vi "Semaphore.vi"() -> ()   [LabVIEW 2020]
panel:
  out "Read":i32
  out "Write":i32
  in  "stop":bool
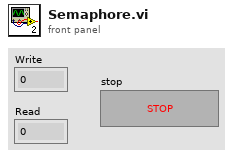
[diagram p1: front panel]
types:
  T1 = typedef "Semaphore RefNum" = refnum<k1>
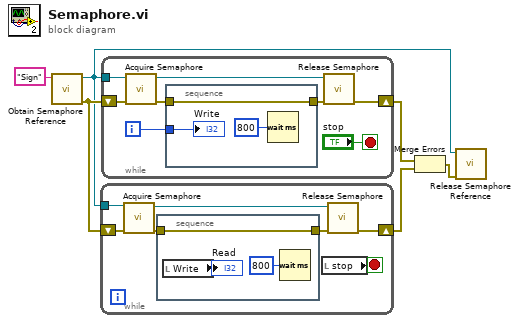
[diagram p0: block diagram]
diagram:
  n1 = call <vilib>:"Obtain Semaphore Reference.vi"("name (unnamed)"="Sign") -> ("error out"=w5:errorcluster, "semaphore"=w4:T1)  [unwired: 4 in, 1 out]
  n2 = while {
    tunnel: w4 -> [w13]
    shift-right: [w7] -> w2
    shift-left: w5 -> [w12]
    stop <- w11 stop-if-true
    n3 = call <vilib>:"Acquire Semaphore.vi"("error in (no error)"=w12, "semaphore"=w13) -> ("error out"=w10:errorcluster, "semaphore out"=w8:T1)  [unwired: 3 in, 1 out]
    n4 = stacked-sequence {
      tunnel: [w16] -> w9
      tunnel: w10 -> [w16]
      frame #0 {
        n5 = local read "Write"() -> (→"Read":i32)
        n6 = Wait (ms)(milliseconds to wait=u32 800) -> ()  [unwired: 1 out]
      }
    }
    n7 = local read "stop"() -> (w11:bool)
    n8 = call <vilib>:"Release Semaphore.vi"("error in (no error)"=w9, "semaphore"=w8) -> ("error out"=w7:errorcluster)  [unwired: 4 in, 1 out]
  }
  n9 = while {
    tunnel: w4 -> [w24]
    shift-right: [w17] -> w3
    shift-left: w5 -> [w23]
    i -> [w19]
    stop <- "stop" stop-if-true
    n10 = call <vilib>:"Acquire Semaphore.vi"("error in (no error)"=w23, "semaphore"=w24) -> ("error out"=w21:errorcluster, "semaphore out"=w18:T1)  [unwired: 3 in, 1 out]
    n11 = stacked-sequence {
      tunnel: w21 -> [w27]
      tunnel: [w27] -> w20
      tunnel: w19 -> [w26]
      frame #0 {
        n12 = Wait (ms)(milliseconds to wait=u32 800) -> ()  [unwired: 1 out]
        "Write" <- w26
      }
    }
    n13 = call <vilib>:"Release Semaphore.vi"("error in (no error)"=w20, "semaphore"=w18) -> ("error out"=w17:errorcluster)  [unwired: 4 in, 1 out]
  }
  n14 = Merge Errors(w3, w2) -> (w1:errorcluster)
  n15 = call <vilib>:"Release Semaphore Reference.vi"("error in (no error)"=w1, "semaphore"=w4) -> ()  [unwired: 8 in, 2 out]
